vi "ConfigureCamera.vi"(8 "error in (no error)":errorcluster, 10 "CameraVideoMode":u32, 11 "Refnum in":T1) -> (0 "error out":errorcluster, 3 "Refnum out":T1)   [LabVIEW 2017]
uses:
  <vilib>/userdefined/High Color/IMAQdx.ctl
  <resource>/objmgr/imaqdx.rc
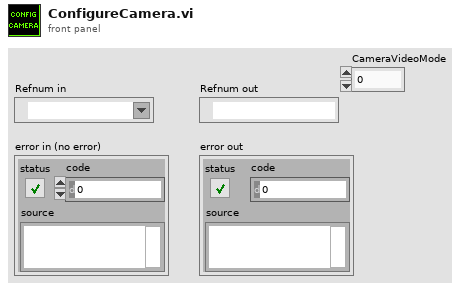
[diagram p1: front panel]
types:
  T1 = typedef "IMAQdx.ctl" = refnum<k21>
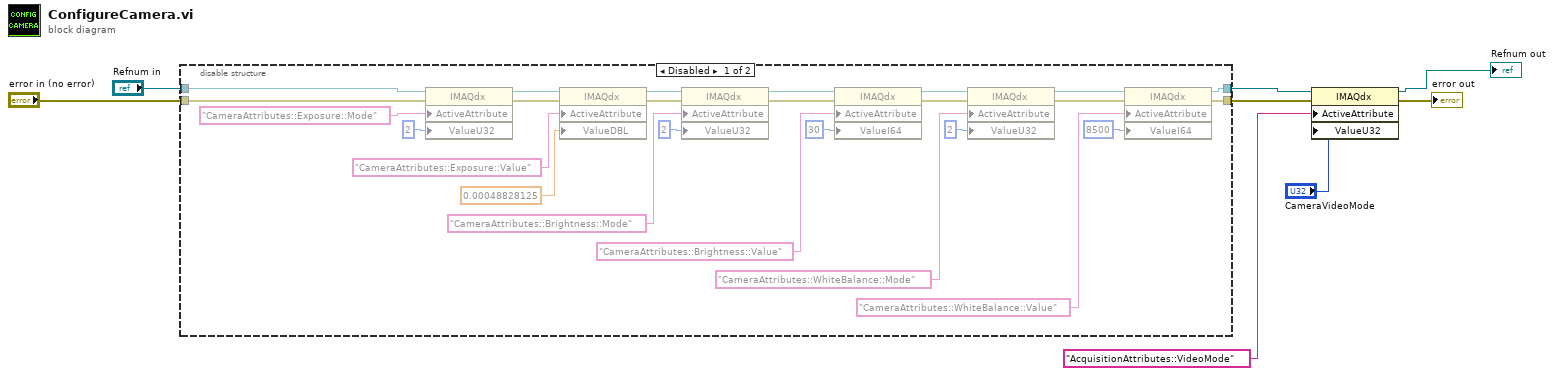
[diagram p0: block diagram]
diagram:
  n1 = disable-structure shown="Disabled" {
    disable-tunnel: "error in (no error)" -> [w34 w35]
    disable-tunnel: "Refnum in" -> [w33 w36]
    disable-tunnel: [w32 w35] -> w4
    disable-tunnel: [w31 w36] -> w3
    frame Disabled {
      n2 = property class="IMAQdx"(reference=w33, error in=w34, "ActiveAttribute"="CameraAttributes::Exposure::Mode", "ValueU32"=u32 2) -> (reference out=w13:T1, error out=w14:errorcluster)
      n3 = property class="IMAQdx"(reference=w13, error in=w14, "ActiveAttribute"="CameraAttributes::Exposure::Value", "ValueDBL"=0.00048828125) -> (reference out=w20:T1, error out=w21:errorcluster)
      n4 = property class="IMAQdx"(reference=w20, error in=w21, "ActiveAttribute"="CameraAttributes::Brightness::Mode", "ValueU32"=u32 2) -> (reference out=w17:T1, error out=w18:errorcluster)
      n5 = property class="IMAQdx"(reference=w17, error in=w18, "ActiveAttribute"="CameraAttributes::Brightness::Value", "ValueI64"=i64 30) -> (reference out=w26:T1, error out=w27:errorcluster)
      n6 = property class="IMAQdx"(reference=w26, error in=w27, "ActiveAttribute"="CameraAttributes::WhiteBalance::Mode", "ValueU32"=u32 2) -> (reference out=w24:T1, error out=w25:errorcluster)
      n7 = property class="IMAQdx"(reference=w24, error in=w25, "ActiveAttribute"="CameraAttributes::WhiteBalance::Value", "ValueI64"=i64 8500) -> (reference out=w31:T1, error out=w32:errorcluster)
    }
    frame Enabled {
    }
  }
  n8 = property class="IMAQdx"(reference=w3, error in=w4, "ActiveAttribute"="AcquisitionAttributes::VideoMode", "ValueU32"="CameraVideoMode") -> (reference out=→"Refnum out":T1, error out=→"error out":errorcluster)
